vi "LCOS Pattern Display_red.vi"() -> ()   [LabVIEW 2011]
uses:
  <vilib>/Utility/miscctls.llb/LVRectTypeDef.ctl
  LCOS Pattern Display Actions.ctl
  <vilib>/vision/Image Controls.llb/IMAQ Image.ctl
panel:
  out "Image":T1(plugin-control)
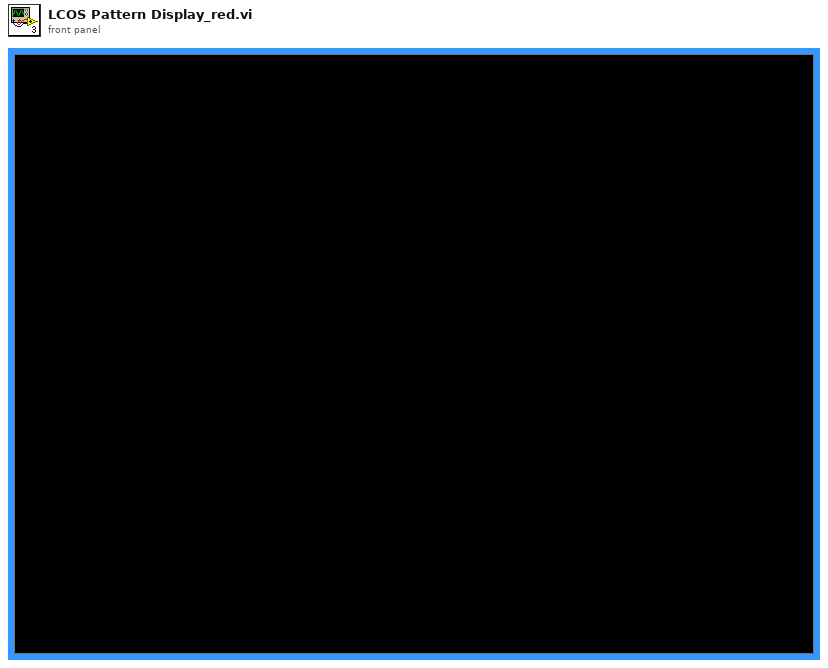
[diagram p1: front panel]
types:
  T1 = typedef "IMAQ Image.ctl" = refnum<image>
  T2 = typedef "LCOS Pattern Display Actions.ctl" = enum16{"Init", "Idle", "Update", "Exit"}
  T3 = cluster{"LCOS Pattern Display Actions":T2, "Data":variant}
  T4 = typedef "LVRectTypeDef.ctl" = cluster{"Left":i16, "Top":i16, "Right":i16, "Bottom":i16}
  T5 = typedef "LVAllMonitorsDisplayTypeDef.ctl" = cluster{"Bounds":cluster{"Left":i16, "Top":i16, "Right":i16, "Bottom":i16}, "Depth":i16}[]
  T6 = cluster{"Bounds":cluster{"Left":i16, "Top":i16, "Right":i16, "Bottom":i16}, "Depth":i16}
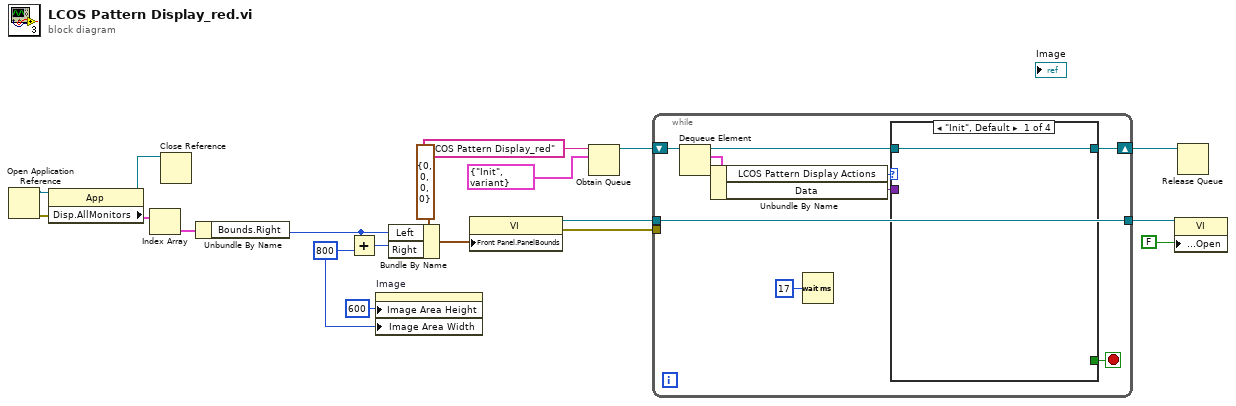
[diagram p0: block diagram]
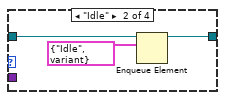
[diagram p2: hidden frame]
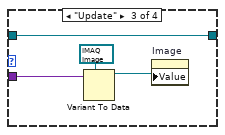
[diagram p3: hidden frame]
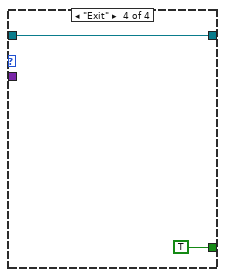
[diagram p4: hidden frame]
diagram:
  w16 = u32 800 ("y")
  n1 = Open Application Reference() -> (0:w3:errorcluster, 3:w6:refnum<vi>)  [unwired: 4 in]
  n2 = property class="App"(reference=w6, error in=w3) -> (reference out=w5:refnum<vi>, "Disp.AllMonitors"=w4:T5)  [unwired: 1 out]
  n3 = Index Array(array=w4) -> (element=w2:T6)  [unwired: 1 in]
  n4 = Close Reference(reference=w5) -> ()  [unwired: 1 in, 1 out]
  n5 = Unbundle By Name(w2) -> ("Bounds.Right"=w1:i16)
  n6 = Add(x=w1, y=w16) -> (x+y=w18:u32)
  n7 = property on="Image" class="ImageControl"("Image Area Height"=u32 600 ("Image Area:Size:Height"), "Image Area Width"=w16) -> ()  [unwired: 2 in, 2 out]
  n8 = Bundle By Name(cluster=T4 {"Left"=0, "Top"=0, "Right"=0, "Bottom"=0} ("Front Panel Window:Panel Bounds"), "Left"=w1, "Right"=w18) -> (w17:T4)
  n9 = property class="VI"("Front Panel.PanelBounds"=w17) -> (reference out=w10:refnum<vi>, error out=w14:errorcluster)  [unwired: 2 in]
  n10 = Obtain Queue(name (unnamed)="LCOS Pattern Display_red", element data type=T3 {"LCOS Pattern Display Actions"=enum."Init", "Data"=variant}) -> (queue out=w12:refnum<queue>)  [unwired: 3 in, 2 out]
  n11 = while {
    tunnel: w14 -> [_]
    shift-right: [w23] -> w7
    shift-left: w12 -> [w28]
    tunnel: w10 -> [w22]
    tunnel: [w22] -> w8
    stop <- w25 stop-if-true
    n12 = Dequeue Element(queue=w28) -> (queue out=w24:refnum<queue>, element=w27:T3)  [unwired: 2 in, 2 out]
    n13 = Unbundle By Name(w27) -> ("LCOS Pattern Display Actions"=w26:T2, "Data"=w20:variant)
    n14 = Wait (ms)(milliseconds to wait=u32 17) -> ()  [unwired: 1 out]
    n15 = case shown="\"Init\", Default" w26 {
      tunnel: [_ _ _ TRUE] -> w25
      tunnel: w24 -> [w29 w32 w34 w37]
      tunnel: [w29 w31 w34 w37] -> w23
      tunnel: w20 -> [_ _ w36 _]
      frame "Init", Default {
      }
      frame "Idle" {
        n16 = Enqueue Element(queue=w32, element=T3 {"LCOS Pattern Display Actions"=enum."Idle", "Data"=variant}) -> (queue out=w31:refnum<queue>)  [unwired: 2 in, 2 out]
      }
      frame "Update" {
        n17 = Variant To Data(type=T1 refnum ("Image"), Variant=w36) -> (data=w33:T1)  [unwired: 1 in, 1 out]
        n18 = property on="Image" class="ImageControl"("Value"=w33) -> ()  [unwired: 2 in, 2 out]
      }
      frame "Exit" {
      }
    }
  }
  n19 = property class="VI"(reference=w8, "Front Panel.Open"=FALSE ("Front Panel Window:Open")) -> ()  [unwired: 1 in, 2 out]
  n20 = Release Queue(queue=w7) -> ()  [unwired: 2 in, 3 out]
